vi "Integral of Polynomial over [a,b].vi"(9 "b":dbl, 10 "a":dbl, 11 "P(x)":dbl[](array[numeric])) -> (0 "error":i32, 3 "integral of P(x)":dbl)   [LabVIEW 2024, in "NI_AALPro.lvlib"]
doc: "<p>Integrates the real polynomial <strong>P(x)</strong> over the interval <strong>a</strong> and <strong>b</strong> define. Integrating a polynomial over an interval [a,b] is the same as calculating the definite integral of the polynomial.</p>"
uses:
  NI_AALPro.lvlib
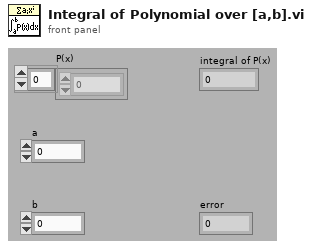
[diagram p1: front panel]
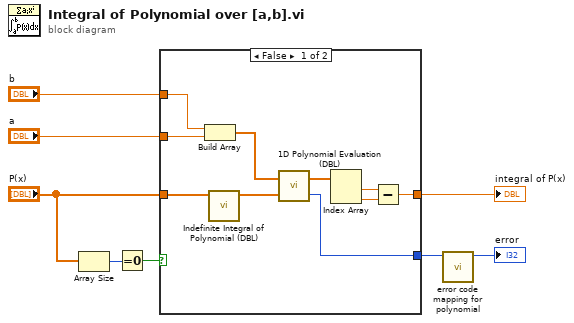
[diagram p0: block diagram]
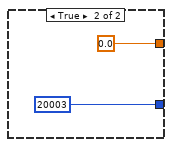
[diagram p2: hidden frame]
diagram:
  n1 = Array Size(array="P(x)") -> (size(s)=w7:i32)
  n2 = Equal To 0?(x=w7) -> (x = 0?=w3:bool)
  n3 = case shown="False" w3 {
    tunnel: "P(x)" -> [w18 _]
    tunnel: "b" -> [w17 _]
    tunnel: "a" -> [w16 _]
    tunnel: [w11 0.0] -> w4
    tunnel: [w9 20003 ("empty array")] -> w2
    frame False {
      n4 = Build Array(w17, w16) -> (w10:dbl[])
      n5 = call "Indefinite Integral of Polynomial (DBL).vi"("P(x)"=w18) -> ("Indefinite Integral of P(x)"=w15:dbl[])  [unwired: 9 in, 1 out]
      n6 = call "1D Polynomial Evaluation (DBL).vi"("P(x)"=w15, "A"=w10) -> ("error"=w9:i32, "P(A)"=w14:dbl[])
      n7 = Index Array(array=w14) -> (element #1=w12:dbl, element #2=w13:dbl)  [unwired: 2 in]
      n8 = Subtract(x=w12, y=w13) -> (x-y=w11:dbl)
    }
    frame True {
    }
  }
  "integral of P(x)" <- w4
  n9 = call "error code mapping for polynomial.vi"("error in"=w2) -> ("error out"=→"error":i32)  [unwired: 10 in]
